vi "Create Resources.vi"() -> (4 "address space collection":refnum<class "Address Space Collection.lvclass">, 15 "stream session":refnum<class "niUSRP Stream Control (DMA) v1 FPGA.lvclass">)   [LabVIEW 2025, in "niUSRP Stream Control (DMA) v1 FPGA.lvclass"]
uses:
  niUSRP Stream Control (DMA) v1 FPGA.lvclass
  <instrlib>/_niInstr/Instruction Framework/v1/FPGA/Interfaces/Address Space Collection/Address Space Collection.lvclass
  C:/Program Files/NI/LVAddons/niidl/1/instr.lib/_niInstr/Instruction Framework/v1/FPGA/Interfaces/Address Space/Address Space.lvclass
  niUSRP Stream Control (DMA) v1 FPGA.lvclass/niUSRP Stream Control (DMA) v1 FPGA.ctl
  <instrlib>/_niInstr/Instruction Framework/v1/FPGA/Helper Classes/Single Address Space Collection/Single Address Space Collection.lvclass
  C:/Program Files/NI/LVAddons/niidl/1/instr.lib/_niInstr/Instruction Framework/v1/FPGA/Interfaces/Address Space Collection/Address Space Collection.lvclass
  <vilib>/rvi/DataTransferAndStorage/Container/Common/niFpgaContainerGetUniqueNameForEmu.vi
  <vilib>/rvi/DataTransferAndStorage/Container/Common/niFpgaContainerSetEmuInfo.vi
  <vilib>/rvi/eio/common/nirviEmuReportErrorAndStop.vi
  <vilib>/rvi/LocalResourceManager/LocalResourceManager.xnode
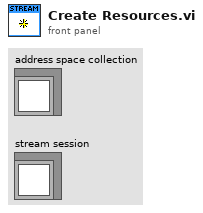
[diagram p1: front panel]
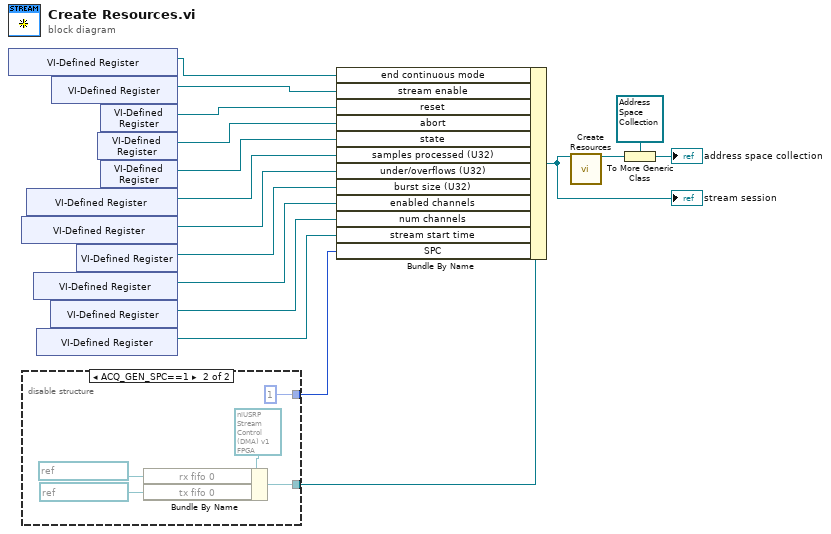
[diagram p0: block diagram]
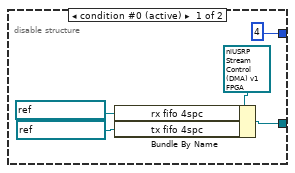
[diagram p2: hidden frame]
diagram:
  n1 = xnode "VI-Defined Register"() -> ("Register Out"=w2:refnum<k21>)
  n2 = xnode "VI-Defined Register"() -> ("Register Out"=w12:refnum<k21>)
  n3 = disable-structure shown="ACQ_GEN_SPC==1" {
    disable-tunnel: [w19 w26] -> w4
    disable-tunnel: [u8 4 ("stream regs.SPC") u8 1 ("stream regs.SPC")] -> w3
    frame condition #0 (active) {
      n4 = Bundle By Name(cluster=refnum<class "niUSRP Stream Control (DMA) v1 FPGA.lvclass"> refnum ("niUSRP Stream Control (DMA) v1 FPGA.lvclass"), "rx fifo 4spc"=refnum<k21> "Rx Stream 0" ("rx fifo"), "tx fifo 4spc"=refnum<k21> "Tx Stream 0" ("tx fifo")) -> (w19:refnum<class "niUSRP Stream Control (DMA) v1 FPGA.lvclass">)
    }
    frame condition #1 {
      n5 = Bundle By Name(cluster=refnum<class "niUSRP Stream Control (DMA) v1 FPGA.lvclass"> refnum ("niUSRP Stream Control (DMA) v1 FPGA.lvclass"), "rx fifo 0"=refnum<k21> "Rx Stream 0" ("rx fifo"), "tx fifo 0"=refnum<k21> "Tx Stream 0" ("tx fifo")) -> (w26:refnum<class "niUSRP Stream Control (DMA) v1 FPGA.lvclass">)
    }
  }
  n6 = xnode "VI-Defined Register"() -> ("Register Out"=w11:refnum<k21>)
  n7 = xnode "VI-Defined Register"() -> ("Register Out"=w6:refnum<k21>)
  n8 = xnode "VI-Defined Register"() -> ("Register Out"=w1:refnum<k21>)
  n9 = xnode "VI-Defined Register"() -> ("Register Out"=w5:refnum<k21>)
  n10 = xnode "VI-Defined Register"() -> ("Register Out"=w14:refnum<k21>)
  n11 = xnode "VI-Defined Register"() -> ("Register Out"=w13:refnum<k21>)
  n12 = xnode "VI-Defined Register"() -> ("Register Out"=w10:refnum<k21>)
  n13 = xnode "VI-Defined Register"() -> ("Register Out"=w8:refnum<k21>)
  n14 = xnode "VI-Defined Register"() -> ("Register Out"=w9:refnum<k21>)
  n15 = Bundle By Name(cluster=w4, "end continuous mode"=w2, "stream enable"=w14, "reset"=w8, "abort"=w10, "state"=w9, "samples processed (U32)"=w11, "under/overflows (U32)"=w12, "burst size (U32)"=w13, "enabled channels"=w6, "num channels"=w5, "stream start time"=w1, "SPC"=w3) -> (w7:refnum<class "niUSRP Stream Control (DMA) v1 FPGA.lvclass">)
  "stream session" <- w7
  n16 = call <instrlib>:"Create Resources.vi"("address space"=w7) -> ("single address space collection"=w15:refnum<class "Single Address Space Collection.lvclass">)  [unwired: 14 in]
  n17 = To More Generic Class(target class=refnum<class "Address Space Collection.lvclass"> refnum ("collection"), reference=w15) -> (generic class reference=→"address space collection":refnum<class "Address Space Collection.lvclass">)
